vi "ParseTokens.vi"(8 "error in (no error)":errorcluster, 11 "PathTokenizer in":refnum<class "PathTokenizer.lvclass">) -> (0 "error out":errorcluster, 3 "PathTokenizer out":refnum<class "PathTokenizer.lvclass">)   [LabVIEW 2019, in "PathTokenizer.lvclass"]
doc: "This will tokenize the path data from the \"d\" attribute of a path object of a scalable vector graphics file. It will separate the data into individual, explicit path commands. \n\nExample:\nM 1.1 2.1 L 3.1 4.1 5.1 6.1\nwill get turned into\nM 1.1 2.1\nL 3.1 4.1\nL 5.1 6.1\nWhich can then be easily parsed."
uses:
  PathTokenizer.lvclass
  PathTokenizer.lvclass/PathTokenizer.ctl
  NextCommand.ctl
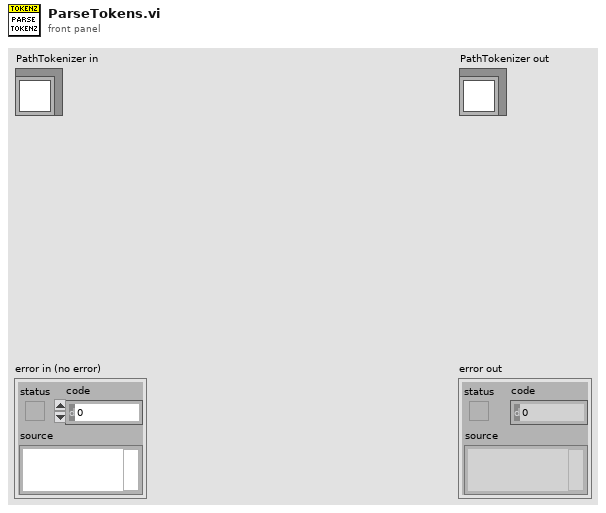
[diagram p1: front panel]
types:
  T1 = typedef "PathTokenizer.lvclass/NextCommand.ctl" = enum16{"Get Coordinate", "Check Explicit", "Check End", "Update Coord Count", "Get Command", "Exit"}
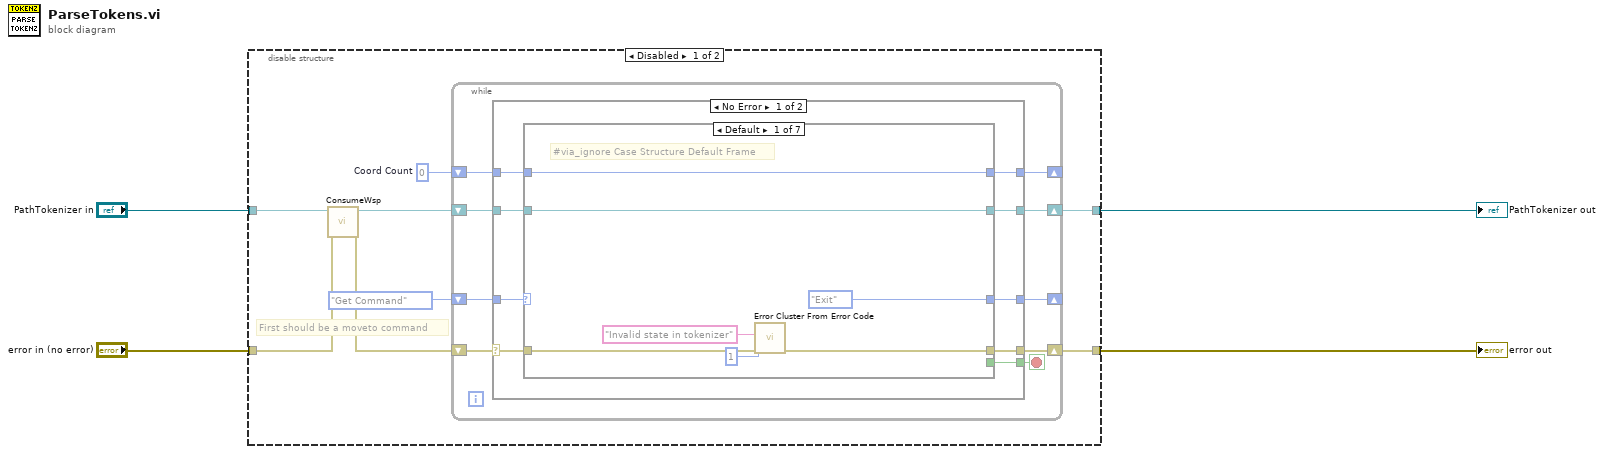
[diagram p0: block diagram]
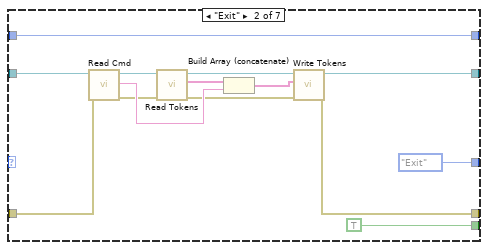
[diagram p2: hidden frame]
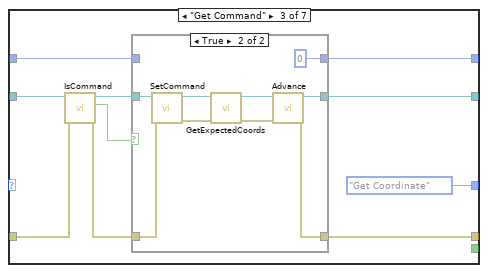
[diagram p3: hidden frame]
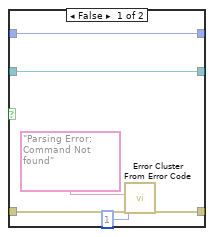
[diagram p4: hidden frame]
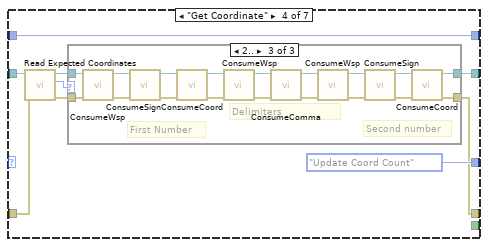
[diagram p5: hidden frame]
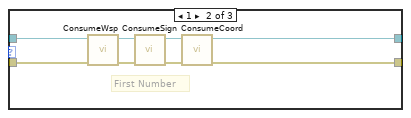
[diagram p7: hidden frame]
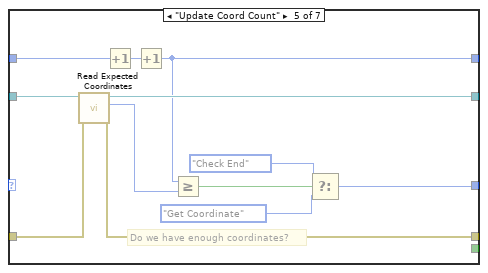
[diagram p8: hidden frame]
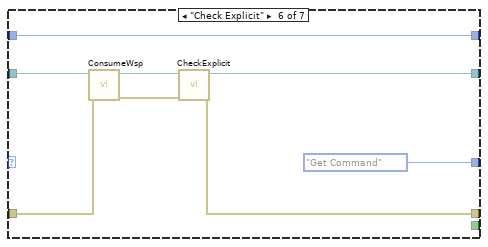
[diagram p9: hidden frame]
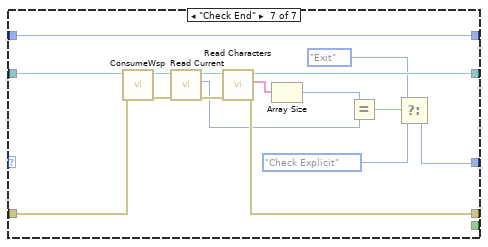
[diagram p10: hidden frame]
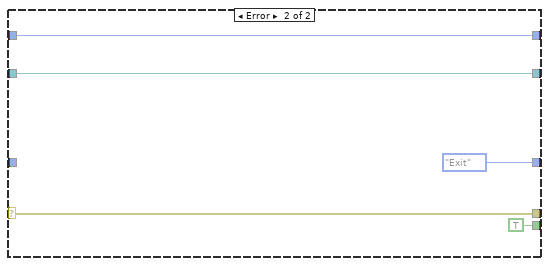
[diagram p11: hidden frame]
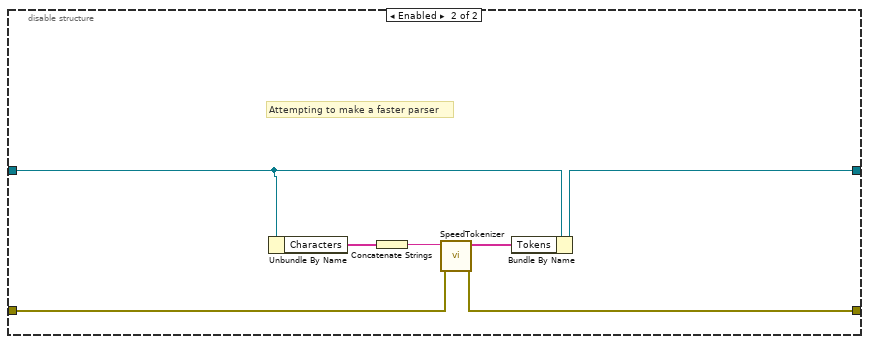
[diagram p12: hidden frame]
diagram:
  n1 = disable-structure shown="Disabled" {
    disable-tunnel: "PathTokenizer in" -> [w12 w155]
    disable-tunnel: [w10 w157] -> w3
    disable-tunnel: [w9 w161] -> w2
    disable-tunnel: "error in (no error)" -> [w8 w158]
    frame Disabled {
      w5 = 0  # Coord Count
      # "First should be a moveto command"
      n2 = call "ConsumeWsp.vi"("error in (no error)"=w8, "PathTokenizer in"=w12) -> ("error out"=w7:errorcluster, "PathTokenizer out"=w11:refnum<class "PathTokenizer.lvclass">)  [unwired: 8 in]
      n3 = while {
        shift-right: [w21] -> w10
        shift-left: w7 -> [w13]
        shift-right: [w19] -> w9
        shift-left: w11 -> [w20]
        shift-right: [w17] -> _
        shift-left: NextCommand."Get Command" -> [w18]
        shift-right: [w14] -> _
        shift-left: w5 -> [w15]
        stop <- w16 stop-if-true
        n4 = case shown="No Error" w13 {
          selector: w13 -> [w22 w151]
          tunnel: [w30 w151] -> w21
          tunnel: w20 -> [w29 w154]
          tunnel: [w28 w154] -> w19
          tunnel: w18 -> [w27 _]
          tunnel: [w26 NextCommand."Exit"] -> w17
          tunnel: [w25 TRUE] -> w16
          tunnel: w15 -> [w24 w153]
          tunnel: [w23 w153] -> w14
          frame No Error {
            n5 = case shown="Default" w27 {
              tunnel: w22 -> [w33 w38 w59 w78 w115 w131 w147]
              tunnel: [w34 w39 w56 w83 w116 w127 w136] -> w30
              tunnel: w29 -> [w37 w47 w60 w80 w124 w132 w148]
              tunnel: [w37 w45 w54 w84 w123 w129 w146] -> w28
              tunnel: [NextCommand."Exit" NextCommand."Exit" NextCommand."Get Coordinate" NextCommand."Update Coord Count" w120 NextCommand."Get Command" w139] -> w26
              tunnel: [_ TRUE _ _ _ _ _] -> w25
              tunnel: w24 -> [w35 w49 w53 w82 w125 w133 w149]
              tunnel: [w35 w49 w52 w82 w117 w133 w149] -> w23
              frame Default {
                # "#via_ignore Case Structure Default Frame"
                n6 = call <vilib>:"Error Cluster From Error Code.vi"("error in (no error)"=w33, "error message (\"\")"="Invalid state in tokenizer" ("error message (\"\")"), "error code (0)"=1) -> ("error out"=w34:errorcluster)  [unwired: 6 in]
              }
              frame "Exit" {
                n7 = call "Read Cmd.vi"("error in (no error)"=w38, "PathTokenizer in"=w47) -> ("error out"=w40:errorcluster, "Cmd"=w43:string, "PathTokenizer out"=w48:refnum<class "PathTokenizer.lvclass">)  [unwired: 7 in]
                n8 = call "Read Tokens.vi"("error in (no error)"=w40, "PathTokenizer in"=w48) -> ("error out"=w41:errorcluster, "Tokens"=w44:string[], "PathTokenizer out"=w46:refnum<class "PathTokenizer.lvclass">)  [unwired: 7 in]
                n9 = Build Array (concatenate)(w44, w43) -> (w42:string[])
                n10 = call "Write Tokens.vi"("error in (no error)"=w41, "Tokens"=w42, "PathTokenizer in"=w46) -> ("error out"=w39:errorcluster, "PathTokenizer out"=w45:refnum<class "PathTokenizer.lvclass">)  [unwired: 7 in]
              }
              frame "Get Command" {
                n11 = call "IsCommand.vi"("error in (no error)"=w59, "PathTokenizer in"=w60) -> ("error out"=w57:errorcluster, "Is Command"=w55:bool, "PathTokenizer out"=w58:refnum<class "PathTokenizer.lvclass">)  [unwired: 7 in]
                n12 = case shown="True" w55 {
                  tunnel: w58 -> [w67 w76]
                  tunnel: [w67 w74] -> w54
                  tunnel: [w66 w73] -> w56
                  tunnel: w57 -> [w65 w75]
                  tunnel: w53 -> [w64 _]
                  tunnel: [w64 0] -> w52
                  frame False {
                    n13 = call <vilib>:"Error Cluster From Error Code.vi"("error in (no error)"=w65, "error message (\"\")"="Parsing Error: Command Not found" ("error message (\"\")"), "error code (0)"=1) -> ("error out"=w66:errorcluster)  [unwired: 6 in]
                  }
                  frame True {
                    n14 = call "SetCommand.vi"("error in (no error)"=w75, "PathTokenizer in"=w76) -> ("error out"=w69:errorcluster, "PathTokenizer out"=w70:refnum<class "PathTokenizer.lvclass">)  [unwired: 8 in]
                    n15 = call "GetExpectedCoords.vi"("error in (no error)"=w69, "PathTokenizer in"=w70) -> ("error out"=w68:errorcluster, "PathTokenizer out"=w71:refnum<class "PathTokenizer.lvclass">)  [unwired: 8 in]
                    n16 = call "Advance.vi"("error in (no error)"=w68, "PathTokenizer in"=w71) -> ("error out"=w73:errorcluster, "PathTokenizer out"=w74:refnum<class "PathTokenizer.lvclass">)  [unwired: 8 in]
                  }
                }
              }
              frame "Get Coordinate" {
                n17 = call "Read Expected Coordinates.vi"("error in (no error)"=w78, "PathTokenizer in"=w80) -> ("error out"=w79:errorcluster, "Expected Coordinates"=w77:i32, "PathTokenizer out"=w81:refnum<class "PathTokenizer.lvclass">)  [unwired: 7 in]
                n18 = case shown="2.." w77 {
                  tunnel: w79 -> [w87 w90 w113]
                  tunnel: [w86 w88 w101] -> w84
                  tunnel: [w87 w89 w97] -> w83
                  tunnel: w81 -> [w86 w91 w96]
                  frame 0, Default {
                    # "#via_ignore Case Structure Default Frame"
                  }
                  frame 1 {
                    # "First Number"
                    n19 = call "ConsumeWsp.vi"("error in (no error)"=w90, "PathTokenizer in"=w91) -> ("error out"=w94:errorcluster, "PathTokenizer out"=w95:refnum<class "PathTokenizer.lvclass">)  [unwired: 8 in]
                    n20 = call "ConsumeSign.vi"("error in (no error)"=w94, "PathTokenizer in"=w95) -> ("error out"=w92:errorcluster, "PathTokenizer out"=w93:refnum<class "PathTokenizer.lvclass">)  [unwired: 8 in]
                    n21 = call "ConsumeCoord.vi"("error in (no error)"=w92, "PathTokenizer in"=w93) -> ("error out"=w89:errorcluster, "PathTokenizer out"=w88:refnum<class "PathTokenizer.lvclass">)  [unwired: 8 in]
                  }
                  frame 2.. {
                    # "Second number"
                    # "Delimiters"
                    # "First Number"
                    n22 = call "ConsumeWsp.vi"("error in (no error)"=w113, "PathTokenizer in"=w96) -> ("error out"=w111:errorcluster, "PathTokenizer out"=w112:refnum<class "PathTokenizer.lvclass">)  [unwired: 8 in]
                    n23 = call "ConsumeSign.vi"("error in (no error)"=w111, "PathTokenizer in"=w112) -> ("error out"=w109:errorcluster, "PathTokenizer out"=w110:refnum<class "PathTokenizer.lvclass">)  [unwired: 8 in]
                    n24 = call "ConsumeCoord.vi"("error in (no error)"=w109, "PathTokenizer in"=w110) -> ("error out"=w106:errorcluster, "PathTokenizer out"=w108:refnum<class "PathTokenizer.lvclass">)  [unwired: 8 in]
                    n25 = call "ConsumeWsp.vi"("error in (no error)"=w106, "PathTokenizer in"=w108) -> ("error out"=w105:errorcluster, "PathTokenizer out"=w107:refnum<class "PathTokenizer.lvclass">)  [unwired: 8 in]
                    n26 = call "ConsumeComma.vi"("error in (no error)"=w105, "PathTokenizer in"=w107) -> ("error out"=w100:errorcluster, "PathTokenizer out"=w104:refnum<class "PathTokenizer.lvclass">)  [unwired: 8 in]
                    n27 = call "ConsumeWsp.vi"("error in (no error)"=w100, "PathTokenizer in"=w104) -> ("error out"=w99:errorcluster, "PathTokenizer out"=w103:refnum<class "PathTokenizer.lvclass">)  [unwired: 8 in]
                    n28 = call "ConsumeSign.vi"("error in (no error)"=w99, "PathTokenizer in"=w103) -> ("error out"=w98:errorcluster, "PathTokenizer out"=w102:refnum<class "PathTokenizer.lvclass">)  [unwired: 8 in]
                    n29 = call "ConsumeCoord.vi"("error in (no error)"=w98, "PathTokenizer in"=w102) -> ("error out"=w97:errorcluster, "PathTokenizer out"=w101:refnum<class "PathTokenizer.lvclass">)  [unwired: 8 in]
                  }
                }
              }
              frame "Update Coord Count" {
                # "Do we have enough coordinates?"
                n30 = call "Read Expected Coordinates.vi"("error in (no error)"=w115, "PathTokenizer in"=w124) -> ("error out"=w116:errorcluster, "Expected Coordinates"=w114:i32, "PathTokenizer out"=w123:refnum<class "PathTokenizer.lvclass">)  [unwired: 7 in]
                n31 = Increment(x=w125) -> (x+1=w119:i32)
                n32 = Increment(x=w119) -> (x+1=w117:i32)
                n33 = Greater Or Equal?(x=w117, y=w114) -> (x >= y?=w118:bool)
                n34 = Select(t=NextCommand."Check End", s=w118, f=NextCommand."Get Coordinate") -> (s? t:f=w120:T1)
              }
              frame "Check Explicit" {
                n35 = call "ConsumeWsp.vi"("error in (no error)"=w131, "PathTokenizer in"=w132) -> ("error out"=w128:errorcluster, "PathTokenizer out"=w130:refnum<class "PathTokenizer.lvclass">)  [unwired: 8 in]
                n36 = call "CheckExplicit.vi"("error in (no error)"=w128, "PathTokenizer in"=w130) -> ("error out"=w127:errorcluster, "PathTokenizer out"=w129:refnum<class "PathTokenizer.lvclass">)  [unwired: 8 in]
              }
              frame "Check End" {
                n37 = call "ConsumeWsp.vi"("error in (no error)"=w147, "PathTokenizer in"=w148) -> ("error out"=w137:errorcluster, "PathTokenizer out"=w144:refnum<class "PathTokenizer.lvclass">)  [unwired: 8 in]
                n38 = call "Read Current.vi"("error in (no error)"=w137, "PathTokenizer in"=w144) -> ("error out"=w138:errorcluster, "Current"=w134:i32, "PathTokenizer out"=w143:refnum<class "PathTokenizer.lvclass">)  [unwired: 7 in]
                n39 = call "Read Characters.vi"("error in (no error)"=w138, "PathTokenizer in"=w143) -> ("error out"=w136:errorcluster, "Characters"=w145:string[], "PathTokenizer out"=w146:refnum<class "PathTokenizer.lvclass">)  [unwired: 7 in]
                n40 = Array Size(array=w145) -> (size(s)=w135:i32)
                n41 = Equal?(x=w135, y=w134) -> (x = y?=w142:bool)
                n42 = Select(t=NextCommand."Exit", s=w142, f=NextCommand."Check Explicit") -> (s? t:f=w139:T1)
              }
            }
          }
          frame Error {
          }
        }
      }
    }
    frame Enabled {
      # "Attempting to make a faster parser"
      n43 = Unbundle By Name(w155) -> ("Characters"=w160:string[])
      n44 = Concatenate Strings(w160) -> (w156:string)
      n45 = call "SpeedTokenizer.vi"("error in (no error)"=w158, "string 2"=w156) -> ("error out"=w157:errorcluster, "Array 2"=w159:string[])  [unwired: 8 in]
      n46 = Bundle By Name(cluster=w155, "Tokens"=w159) -> (w161:refnum<class "PathTokenizer.lvclass">)
    }
  }
  "error out" <- w3
  "PathTokenizer out" <- w2
